vi "svl_Check Integration Type.vi"(6 "integration type":T1(ring)=enum."double integration", 7 "reset (in)":bool, 8 "error in (no error)":errorcluster) -> (0 "error out":errorcluster, 2 "parameter has changed":bool)   [LabVIEW 2017, in "SoundVib_Integration.lvlib"]
uses:
  <vilib>/addons/Sound and Vibration/svt_Integration/SoundVib_Integration.lvlib
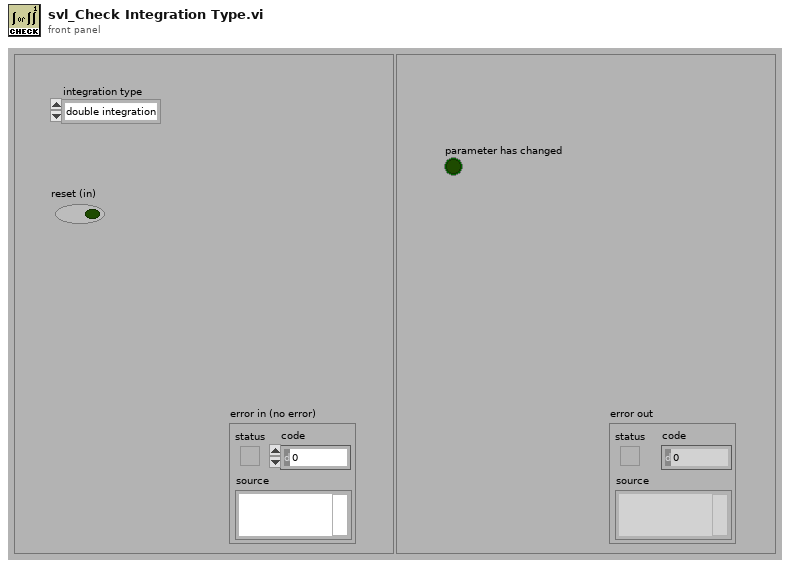
[diagram p1: front panel]
types:
  T1 = enum16{"single integration", "double integration"}
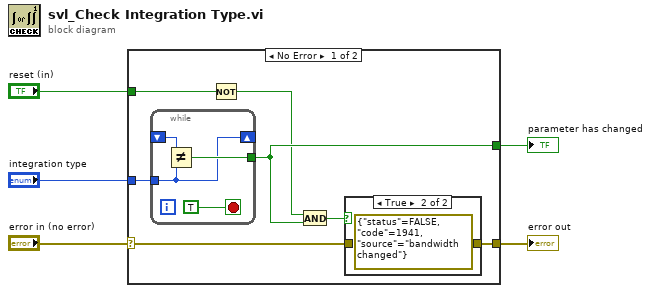
[diagram p0: block diagram]
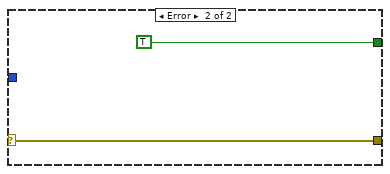
[diagram p3: hidden frame]
diagram:
  n1 = case shown="No Error" "error in (no error)" {
    selector: "error in (no error)" -> [w11 w20]
    tunnel: [w10 w20] -> w4
    tunnel: "integration type" -> [w12 _]
    tunnel: [w8 TRUE] -> w3
    tunnel: "reset (in)" -> [w7 _]
    frame No Error {
      n2 = while {
        tunnel: [w15] -> w8
        tunnel: w12 -> [w13]
        shift-left: _ -> [w14]
        shift-right: [w13] -> _
        stop <- TRUE stop-if-true
        n3 = Not Equal?(x=w14, y=w13) -> (x != y?=w15:bool)
      }
      n4 = Not(x=w7) -> (.not. x?=w6:bool)
      n5 = And(x=w6, y=w8) -> (x .and. y?=w9:bool)
      n6 = case shown="True" w9 {
        tunnel: w11 -> [w17 _]
        tunnel: [w17 errorcluster {"status"=FALSE, "code"=1941, "source"="bandwidth changed"} ("error IO")] -> w10
        frame False {
        }
        frame True {
        }
      }
    }
    frame Error {
    }
  }
  "error out" <- w4
  "parameter has changed" <- w3
